vi "Get Trace.vi"(8 "error in (no error)":errorcluster, 11 "Receiver in":refnum<class "Receiver.lvclass">) -> (0 "error out":errorcluster, 3 "Receiver out":refnum<class "Receiver.lvclass">)   [LabVIEW 2013, in "Receiver.lvlib" / "Receiver.lvclass"]
uses:
  Receiver.lvclass
  Connected Messages/Trace Gotten Msg/Trace Gotten Msg.lvclass
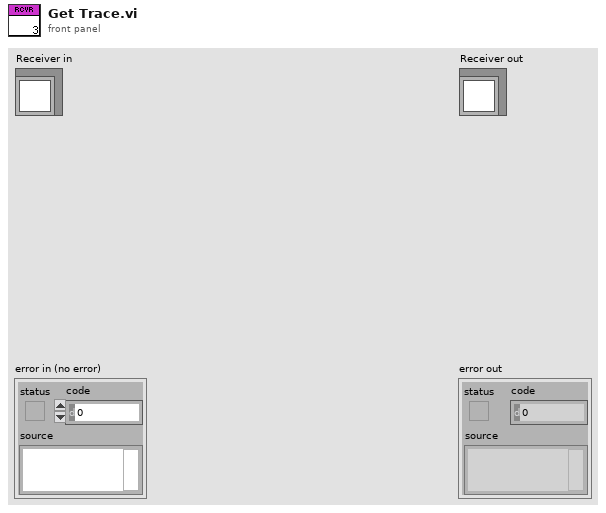
[diagram p1: front panel]
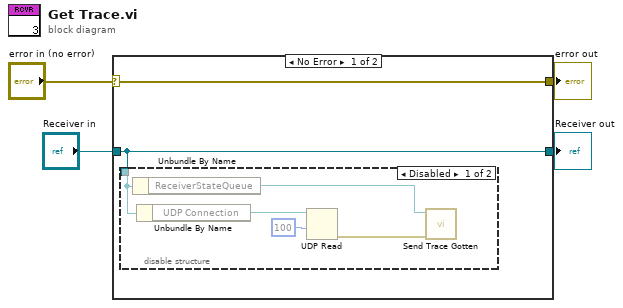
[diagram p0: block diagram]
diagram:
  n1 = case shown="No Error" "error in (no error)" {
    selector: "error in (no error)" -> [w6 w13]
    tunnel: [w6 w13] -> w3
    tunnel: [w5 w12] -> w1
    tunnel: "Receiver in" -> [w5 w12]
    frame No Error {
      n2 = disable-structure shown="Disabled" {
        disable-tunnel: w5 -> [w9 _]
        frame Disabled {
          n3 = Unbundle By Name(w9) -> ("ReceiverStateQueue"=w8:refnum<class "Message Enqueuer.lvclass">)
          n4 = Unbundle By Name(w9) -> ("UDP Connection"=w11:refnum<k16>)
          n5 = UDP Read(connection ID=w11, timeout ms (25000)=100) -> (error out=w7:errorcluster)  [unwired: 2 in, 4 out]
          n6 = call "Send Trace Gotten.vi"("error in (no error)"=w7, "Message Enqueuer"=w8) -> ()  [unwired: 8 in, 2 out]
        }
        frame Enabled {
        }
      }
    }
    frame Error {
    }
  }
  "error out" <- w3
  "Receiver out" <- w1
